vi "Test1_1_ASIC.vi"(4 "Voltages comprobation":dbl[](array[numeric])=[0.05, 0.1, 0.2, 0.5, 0.8, 0.5, 0.6, 0.7, 0.8, 1.0], 7 "Serial Number":string, 8 "error in":errorcluster, 9 "Cycles Burst":i32=10000, 10 "Channels":i32[](array[numeric])=[0, 1, 2, 3, 4, 5, 6], 11 "Instrument VISA in":T1={"AWG VISA"="generadorpulsos", "Oscilloscope  VISA "="Oscilloscope", "Integration Board IP"="172.16.7.43", "connection ID"=refnum, "report out"=refnum, "report file path"=path "C:/Documents and Settings/CTA_LAB01/Desktop/L0_Asic/L0 Asic Test Data"}) -> (0 "error out":errorcluster, 3 "Instrument VISA out":T1={"AWG VISA"="81160A", "Oscilloscope  VISA "="DSO80204B", "Integration Board IP"="172.16.7.43", "connection ID"=refnum, "report out"=refnum, "report file path"=path "C:/Documents and Settings/CTA_LAB01/Desktop/L0_Asic/L0 Asic Test Data"}, 5 "Array":i32[][](array[numeric]))   [LabVIEW 2009]
uses:
  <vilib>/Utility/NIReport.llb/NI_report.lvclass
  <vilib>/Utility/NIReport.llb/HTML/NI_HTML.lvclass
  <instrlib>/Agilent 81150/Agilent 81150.lvlib
  L0_Asic/L0 Asic Test Folder v9/C/Program Files/National Instruments/LabVIEW 2012/instr.lib/Agilent 8000 Series/Agilent 8000 Series.lvlib
  <vilib>/Analysis/NI_AALBase.lvlib
panel:
  in  "Attenuation":i32[](array[numeric])=[0, 4, 10, 12]
  out "Threshold array":i32[](array[numeric])
  out "read buffer 4":string="-1.51468E-08;9.99999E+37;9.99999E+37;1.3964E-09;9.99999E+37;9.99999E+37\n"
  out "report file path":path=path "D:/CTA/Data_test/ASIC/chip_test"
  in  "time to wait":dbl=10.0
  in  "Init values ch":i32[](array[numeric])=[500, 500, 500, 500, 500, 500, 500]
  out "Data output":dbl[][](array[numeric])
  out "time for inner bucle":u32=249
  out "read buffer 3":string
  out "appended array":dbl[](array[numeric])=[1.999998e+38, 0.0, 1.3964e-09, 0.0, 9.99999e+37, 0.0, 9.99999e+37, 0.0, -1.51468e-08, 0.0, 0.0]
  out "points quantity":dbl
  out "Numeric":i32=2147483647
  in  "Save NOW!":bool
  in  "End 2":bool
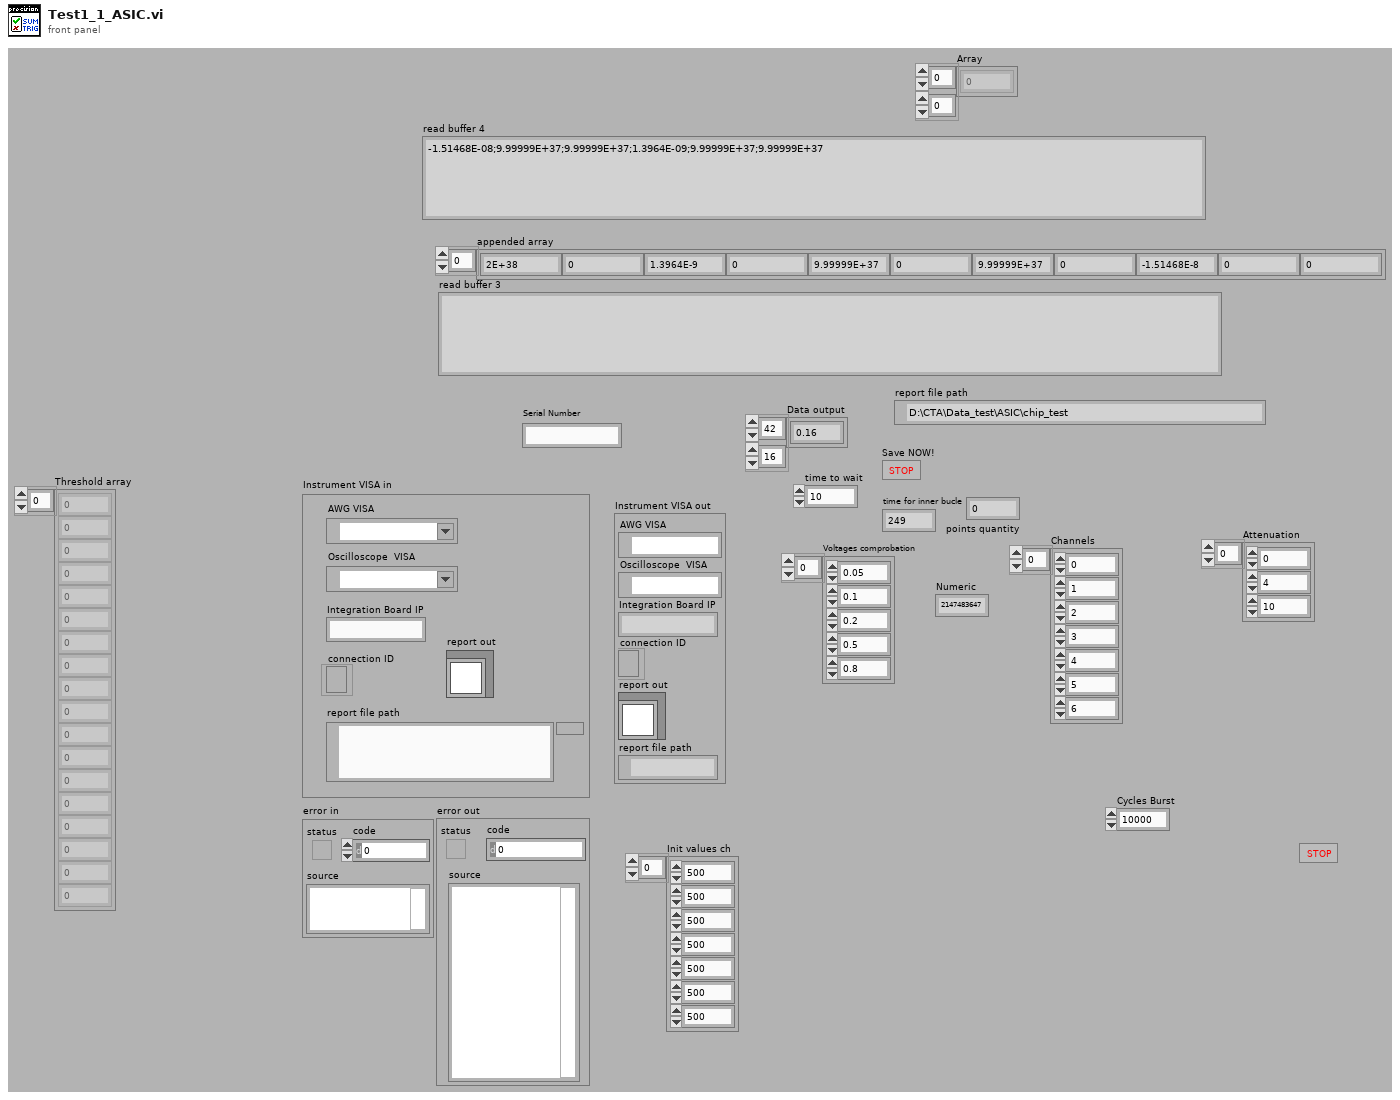
[diagram p1: front panel]
types:
  T1 = cluster{"AWG VISA":refnum<visa-resource-name>, "Oscilloscope  VISA ":refnum<visa-resource-name>, "Integration Board IP":string, "connection ID":refnum<k5>, "report out":refnum<class "NI_report.lvclass">, "report file path":path}
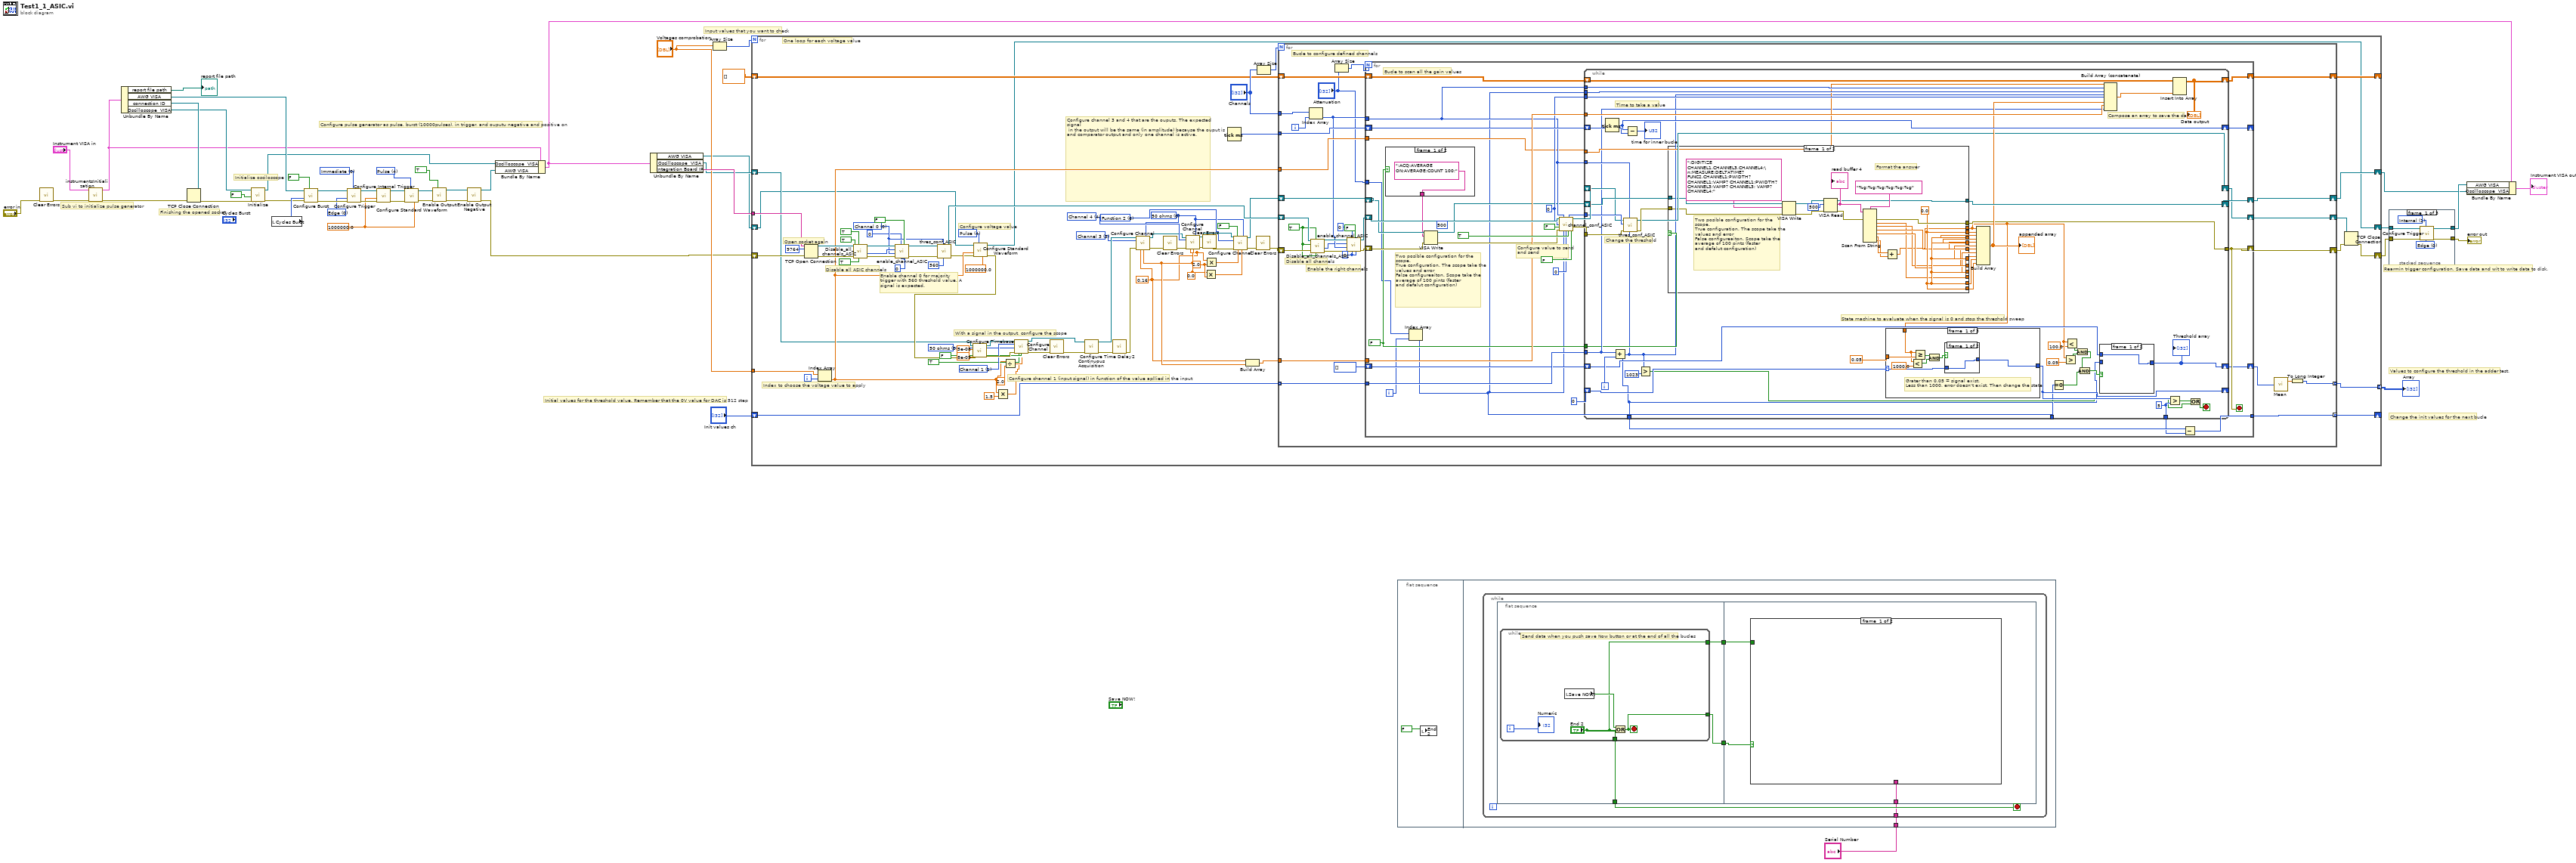
[diagram p0: block diagram]
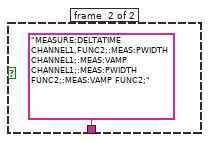
[diagram p2: hidden frame]
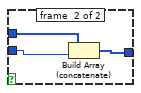
[diagram p3: hidden frame]
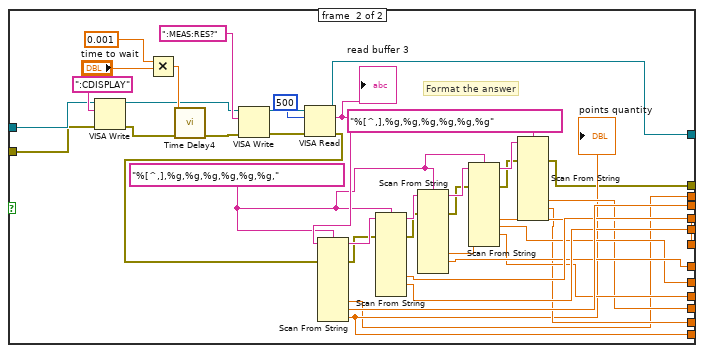
[diagram p4: hidden frame]
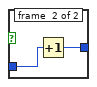
[diagram p5: hidden frame]
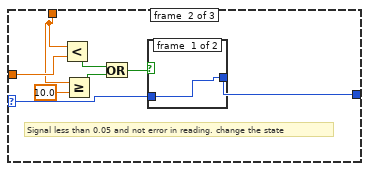
[diagram p6: hidden frame]
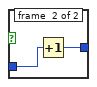
[diagram p7: hidden frame]
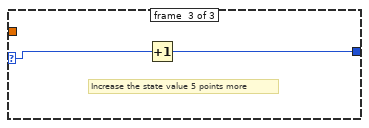
[diagram p8: hidden frame]
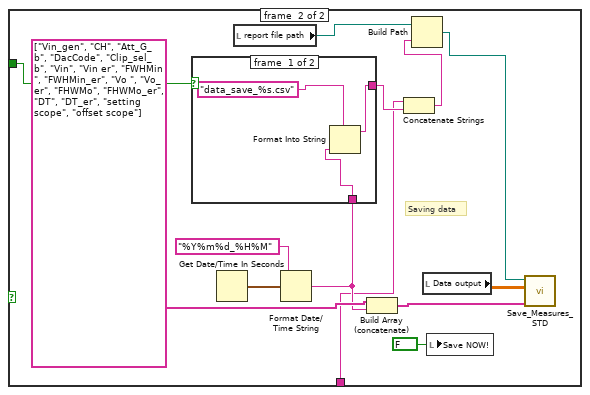
[diagram p9: hidden frame]
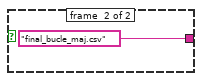
[diagram p10: hidden frame]
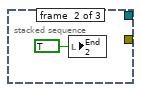
[diagram p11: hidden frame]
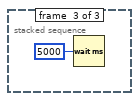
[diagram p12: hidden frame]
diagram:
  w12 = 1000000.0 ("Frequency (1000.0 Hz)")
  w39 = u16 0 items=["Immediate", "Internal", "External", "Software Trigger Function"] ("Trigger Source (0: Immediate)")
  w40 = u16 0 items=["Edge", "Level"] ("Trigger Mode (0: Edge)")
  w44 = u16 4 items=["Sine", "Square", "Ramp Up", "Ramp Down", "Pulse", "Noise", "DC"] ("Waveform (0: Sine)")
  # "Values to configure the threshold in the adder test."
  # "Rearmin trigger configuration. Save data and wit to write data to disk."
  # "Change the init values for the next bucle"
  # "Input values that you want to check"
  # "Initial values for the threshold value. Remember that the 0V value for DAC is 512 step"
  # "Configure pulse generator as pulse, burst (10000pulses), in trigger, and ouputu negative and positive on"
  # "Initialize osciloscope"
  # "Finishing the opened socket"
  # "Sub vi to initialize pulse generator"
  n1 = call <vilib>:"Clear Errors.vi"("error in (no error)"="error in") -> ("error out"=w46:errorcluster)  [unwired: 6 in]
  n2 = call "instrumentsInitialization.vi"("error in"=w46, "Instrument VISA in"="Instrument VISA in") -> ("error out"=w33:errorcluster, "Instrument VISA out"=w24:T1)  [unwired: 8 in]
  n3 = Unbundle By Name(w24) -> ("report file path"=→"report file path":path, "AWG VISA"=w29:refnum<visa-resource-name>, "connection ID"=w34:refnum<k5>, "Oscilloscope  VISA"=w30:refnum<visa-resource-name>)
  n4 = TCP Close Connection(connection ID=w34, error in (no error)=w33) -> (error out=w28:errorcluster)  [unwired: 1 in, 1 out]
  n5 = call "Initialize.vi"("error in (no error)"=w28, "Reset (True)"=FALSE ("ID Query (True)"), "VISA resource name"=w30) -> ("error out"=w8:errorcluster, "VISA resource name out"=w27:refnum<visa-resource-name>)  [unwired: 7 in]
  n6 = local read "Cycles Burst"() -> (w43:i32)
  n7 = call <instrlib>:"Configure Burst.vi"("Enable Burst (F: Disable)"=FALSE, "error in (no error)"=w8, "Burst Count (2)"=w43, "VISA resource name"=w29) -> ("error out"=w42:errorcluster, "VISA resource name out"=w41:refnum<visa-resource-name>)  [unwired: 6 in]
  n8 = call <instrlib>:"Configure Trigger.vi"("Trigger Source (0: Immediate)"=w39, "error in (no error)"=w42, "Trigger Mode (0: Edge)"=w40, "VISA resource name"=w41) -> ("error out"=w38:errorcluster, "VISA resource name out"=w37:refnum<visa-resource-name>)  [unwired: 6 in]
  n9 = call <instrlib>:"Configure Internal Trigger.vi"("error in (no error)"=w38, "Frequency (100000.0 Hz)"=w12, "VISA resource name"=w37) -> ("error out"=w35:errorcluster, "VISA resource name out"=w36:refnum<visa-resource-name>)  [unwired: 7 in]
  n10 = call <instrlib>:"Configure Standard Waveform.vi"("Frequency (1000.0 Hz)"=w12, "Waveform (0: Sine)"=w44, "error in (no error)"=w35, "VISA resource name"=w36) -> ("error out"=w26:errorcluster, "VISA resource name out"=w25:refnum<visa-resource-name>)  [unwired: 6 in]
  n11 = call <instrlib>:"Enable Output.vi"("Enable Output (T: Enable)"=TRUE, "error in (no error)"=w26, "VISA resource name"=w25) -> ("error out"=w11:errorcluster, "VISA resource name out"=w10:refnum<visa-resource-name>)  [unwired: 7 in]
  n12 = call <instrlib>:"Enable Output Negative.vi"("error in (no error)"=w11, "VISA resource name"=w10) -> ("error out"=w2:errorcluster, "VISA resource name out"=w9:refnum<visa-resource-name>)  [unwired: 8 in]
  n13 = Bundle By Name(cluster=w24, "Oscilloscope  VISA"=w27, "AWG VISA"=w9) -> (w7:T1)
  n14 = Unbundle By Name(w7) -> ("AWG VISA"=w5:refnum<visa-resource-name>, "Oscilloscope  VISA"=w6:refnum<visa-resource-name>, "Integration Board IP"=w20:string)
  n15 = Array Size(array="Voltages comprobation") -> (size(s)=w17:i32)
  n16 = for {
    N: w17 -> [_]
    tunnel: w20 -> [w126]
    tunnel: "Voltages comprobation" -> [w125]
    shift-right: [w85] -> _
    shift-left: dbl[][] [] -> [w86]
    shift-right: [w83] -> _
    shift-left: "Init values ch" -> [w84]
    shift-right: [w61] -> w14
    shift-left: w6 -> [w57]
    shift-right: [w127] -> w21
    shift-left: w2 -> [w58]
    shift-right: [w56] -> w13
    shift-left: w5 -> [w50]
    tunnel: [w49] -> w3 mode=indexing
    i -> [w81]
    w62 = 0.16 ("Vertical Range (2.0 V)")
    w63 = 0.0 ("Vertical Offset (0.0 V)")
    w80 = u32 0 ("Clip_sel_b")
    w93 = 2.0 ("y")
    w65 = u32 0 items=["50 ohms", "1 Mohms"] ("Input Impedance (1: 1 Mohms)")
    w73 = u16 0 items=["Channel 0", "Channel 1", "Channel 2", "Channel 3", "Channel 4", "Channel 5", "Channel 6"] ("Channel")
    w113 = u32 0 items=["50 ohms", "1 Mohms"] ("Input Impedance (1: 1 Mohms)")
    w116 = 1 items=["Channel 1"=1, "Channel 2"=2, "Channel 3"=3, "Channel 4"=4] ("Channel (1: Channel 1)")
    w97 = u16 6 items=["Function 1"=5, "Function 2"=6, "Function 3"=7, "Function 4"=8] ("Math Channel (5: Function 1)")
    w64 = 3 items=["Channel 1"=1, "Channel 2"=2, "Channel 3"=3, "Channel 4"=4] ("Channel (1: Channel 1)")
    w111 = 4 items=["Channel 1"=1, "Channel 2"=2, "Channel 3"=3, "Channel 4"=4] ("Channel (1: Channel 1)")
    w123 = u16 4 items=["Sine", "Square", "Ramp Up", "Ramp Down", "Pulse", "Noise", "DC"] ("Waveform (0: Sine)")
    # "Configure channel 3 and 4 that are the ouputs. The expected signal\n in the output will be the same (in amplitude) because the ouput is and comparator output and only one channel is active."
    # "Configure channel 1 (input signal) in function of the value apllied in the input"
    # "With a signal in the output, configure the scope"
    # "Enable channel 0 for majority trigger with 560 threshold value. A signal is expected."
    # "Disable all ASIC channels"
    # "Open socket again"
    # "Configure voltage value"
    # "Index to choose the voltage value to apply"
    # "One loop for each voltage value"
    n17 = TCP Open Connection(address=w126, remote port or service name=u16 9764, error in (no error)=w58) -> (connection ID=w107:refnum<k5>, error out=w106:errorcluster)  [unwired: 2 in]
    n18 = Index Array(array=w125, index=w81) -> (element=w82:dbl)
    n19 = call "Disable_all_channels_ASIC.vi"("CompBuf_en_b"=TRUE, "Att_en_b"=TRUE, "error in"=w106, "Clip_en_b"=TRUE, "connection ID"=w107) -> ("error out"=w105:errorcluster, "id_out"=w103:i32, "connection ID out"=w104:refnum<k5>)  [unwired: 4 in]
    n20 = call "enable_channel_ASIC.vi"("Clip_sel_b"=w80, "maj/sum"=FALSE, "Ib_clipVb"=w80, "Att gain"=u32 0, "error in"=w105, "Channel"=w73, "id_in"=w103, "connection ID"=w104) -> ("error out"=w76:errorcluster, "connection ID out"=w78:refnum<k5>)  [unwired: 1 in, 1 out]
    n21 = call "thres_conf_ASIC.vi"("threshold"=u32 560, "Ring"=w73, "error out 3"=w76, "connection ID"=w78) -> ("error out 2"=w75:errorcluster, "connection ID out"=w77:refnum<k5>)  [unwired: 4 in, 2 out]
    n22 = call <instrlib>:"Configure Standard Waveform.vi"("Frequency (1000.0 Hz)"=1000000.0, "Waveform (0: Sine)"=w123, "error in (no error)"=w75, "Amplitude (1.0 Vpp)"=w82, "VISA resource name"=w50) -> ("error out"=w120:errorcluster, "VISA resource name out"=w56:refnum<visa-resource-name>)  [unwired: 5 in]
    n23 = call "Configure Timebase.vi"("error in (no error)"=w120, "Position (0.0 s)"=8e-09, "Timebase (0.005 s)"=5e-08, "VISA resource name"=w57) -> ("error out"=w117:errorcluster, "VISA resource name out"=w118:refnum<visa-resource-name>)  [unwired: 6 in]
    n24 = Multiply(x=w82, y=1.5) -> (x*y=w94:dbl)
    n25 = Divide(x=w82, y=2.0) -> (x/y=w102:dbl)
    n26 = call "Configure Channel.vi"("VISA resource name"=w118, "Enable Channel (Enable)"=TRUE, "BW Limit 20MHz (Disable)"=FALSE, "Input Impedance (1: 1 Mohms)"=w113, "Channel (1: Channel 1)"=w116, "error in (no error)"=w117, "Vertical Range (2.0 V)"=w94, "Vertical Offset (0.0 V)"=w102) -> ("VISA resource name out"=w53:refnum<visa-resource-name>, "error out"=w115:errorcluster)  [unwired: 6 in]
    n27 = call <vilib>:"Clear Errors.vi"("error in (no error)"=w115) -> ("error out"=w52:errorcluster)  [unwired: 6 in]
    n28 = call "Configure Continuous Acquisition.vi"("error in (no error)"=w52, "VISA resource name"=w53) -> ("error out"=w96:errorcluster, "VISA resource name out"=w66:refnum<visa-resource-name>)  [unwired: 8 in]
    n29 = call "Time Delay2"("error in (no error)"=w96) -> ("error out"=w67:errorcluster)  [unwired: 10 in]
    n30 = call "Configure Channel.vi"("VISA resource name"=w66, "Input Impedance (1: 1 Mohms)"=w65, "Channel (1: Channel 1)"=w64, "error in (no error)"=w67, "Vertical Range (2.0 V)"=w62, "Vertical Offset (0.0 V)"=w63) -> ("VISA resource name out"=w68:refnum<visa-resource-name>, "error out"=w69:errorcluster)  [unwired: 8 in]
    n31 = call <vilib>:"Clear Errors.vi"("error in (no error)"=w69) -> ("error out"=w108:errorcluster)  [unwired: 6 in]
    n32 = call "Configure Channel.vi"("VISA resource name"=w68, "Input Impedance (1: 1 Mohms)"=w65, "Channel (1: Channel 1)"=w111, "error in (no error)"=w108, "Vertical Range (2.0 V)"=w62, "Vertical Offset (0.0 V)"=w63) -> ("VISA resource name out"=w99:refnum<visa-resource-name>, "error out"=w109:errorcluster)  [unwired: 8 in]
    n33 = call <vilib>:"Clear Errors.vi"("error in (no error)"=w109) -> ("error out"=w100:errorcluster)  [unwired: 6 in]
    n34 = Multiply(x=w63, y=w93) -> (x*y=w92:dbl)
    n35 = Multiply(x=w62, y=w93) -> (x*y=w98:dbl)
    n36 = Tick Count (ms)() -> (millisecond timer value=w90:u32)
    n37 = call "Configure Channel.vi"("VISA resource name"=w99, "Enable Channel (Enable)"=FALSE, "Input Impedance (1: 1 Mohms)"=w65, "Channel (1: Channel 1)"=w97, "error in (no error)"=w100, "Vertical Range (2.0 V)"=w98, "Vertical Offset (0.0 V)"=w92) -> ("VISA resource name out"=w60:refnum<visa-resource-name>, "error out"=w101:errorcluster)  [unwired: 7 in]
    n38 = Build Array(w62, w63) -> (w89:dbl[])
    n39 = call <vilib>:"Clear Errors.vi"("error in (no error)"=w101) -> ("error out"=w91:errorcluster)  [unwired: 6 in]
    n40 = Array Size(array="Channels") -> (size(s)=w88:i32)
    n41 = for {
      N: w88 -> [_]
      tunnel: w90 -> [w157]
      tunnel: w89 -> [w156]
      tunnel: "Channels" -> [w155]
      shift-right: [w158] -> w85
      shift-left: w86 -> [w153]
      tunnel: w84 -> [w152] mode=indexing
      tunnel: [w151] -> w83 mode=indexing
      tunnel: w82 -> [w150]
      shift-right: [w149] -> w61
      shift-left: w60 -> [w148]
      shift-right: [w147] -> w59
      shift-left: w91 -> [w144]
      shift-right: [w146] -> w55
      shift-left: w77 -> [w141]
      tunnel: [w130] -> w49 mode=indexing
      i -> [w154]
      w138 = u32 0 ("Ib_clipVb")
      w139 = TRUE ("Att_en_b")
      # "Enable the right channels"
      # "Disable all channels"
      # "Bucle to configure defined channels"
      n42 = Index Array(array=w155, index=w154) -> (element=w136:i32)
      n43 = call "Disable_all_channels_ASIC.vi"("CompBuf_en_b"=w139, "Att_en_b"=w139, "error in"=w144, "Clip_en_b"=w139, "connection ID"=w141) -> ("error out"=w145:errorcluster, "id_out"=w135:i32, "connection ID out"=w142:refnum<k5>)  [unwired: 4 in]
      n44 = Array Size(array="Attenuation") -> (size(s)=w129:i32)
      n45 = call "enable_channel_ASIC.vi"("Clip_sel_b"=w138, "maj/sum"=FALSE, "Ib_clipVb"=w138, "Att gain"=u32 0, "error in"=w145, "Channel"=w136, "id_in"=w135, "connection ID"=w142) -> ("error out"=w143:errorcluster, "connection ID out"=w140:refnum<k5>)  [unwired: 1 in, 1 out]
      n46 = for {
        N: w129 -> [_]
        shift-right: [w185] -> w147
        shift-left: w143 -> [w170]
        shift-right: [w186] -> w158
        shift-left: w153 -> [w193]
        shift-right: [w187] -> w149
        shift-left: w148 -> [w169]
        shift-right: [w179] -> w146
        shift-left: w140 -> [w192]
        tunnel: w156 -> [w190]
        shift-right: [w188] -> _
        shift-left: w157 -> [w189]
        tunnel: w136 -> [w178]
        tunnel: w152 -> [w176]
        tunnel: [w171] -> w151
        tunnel: w150 -> [w174]
        shift-right: [w163] -> w131
        shift-left: i32[] [] -> [w162]
        tunnel: "Attenuation" -> [w161]
        i -> [w160]
        stop <- w185 stop-if-true
        w164 = FALSE
        (unwired) u32 500 ("byte count")
        w180 = u32 0 ("Ib_ClipVb")
        # "Configure value to send and send"
        # "Two posible configuration for the scope. \nTrue configuration. The scope take the values and error\nFalse configureaiton. Scope take the average of 100 pints (faster\nand defalut configuration)"
        # "Bucle to scan all the gain values"
        n47 = case shown="False" w164 {
          tunnel: [":ACQ:AVERAGE ON;AVERAGE:COUNT 100;" ("write buffer") "MEASURE:DELTATIME CHANNEL1,FUNC2;:MEAS:PWIDTH CHANNEL1;:MEAS:VAMP CHANNEL1;:MEAS:PWIDTH FUNC2;:MEAS:VAMP FUNC2;" ("write buffer")] -> w168
          frame #0 {
          }
          frame #1 {
          }
        }
        n48 = Index Array(array=w161, index=w160) -> (element=w159:i32)
        n49 = VISA Write(VISA resource name=w169, write buffer=w168, error in (no error)=w170) -> (VISA resource name out=w166:refnum<visa-resource-name>, error out=w165:errorcluster)  [unwired: 1 out]
        n50 = call "channel_conf_ASIC.vi"("connection ID"=w192, "Ring"=w178, "Clip_sel_b"=w180, "CompBuf_en_b"=FALSE, "error out"=w165, "Att gain"=w159, "Ib_ClipVb"=u32 0, "Clip_en_b"=TRUE, "Att_en_b"=FALSE) -> ("Id out"=w177:i32, "connection ID out"=w167:refnum<k5>, "error out 2"=w182:errorcluster)  [unwired: 2 in, 2 out]
        n51 = while {
          tunnel: w190 -> [w247]
          tunnel: [w230] -> w185
          tunnel: w182 -> [w224]
          tunnel: w180 -> [w228]
          tunnel: w178 -> [w227]
          tunnel: w159 -> [w226]
          tunnel: w178 -> [w222]
          tunnel: w177 -> [w221]
          tunnel: w176 -> [w209]
          shift-right: [w216] -> _
          shift-left: 0 -> [w219]
          tunnel: [w196] -> w173
          tunnel: w174 -> [w217]
          tunnel: [w215] -> w172
          shift-right: [w245] -> w188
          shift-left: w189 -> [w246]
          shift-right: [w243] -> w187
          shift-left: w166 -> [w229]
          shift-right: [w223] -> w179
          shift-left: w167 -> [w214]
          shift-right: [w240] -> w186
          shift-left: w193 -> [w248]
          tunnel: w164 -> [w208]
          shift-right: [w206] -> w163
          shift-left: w162 -> [w205]
          tunnel: w159 -> [w202]
          i -> [w220]
          stop <- w211 stop-if-true
          w215 = 5 ("y")
          # "State machine to evaluate when the signal is 0 and stop the threshold sweep"
          # "Compose an array to save the data"
          # "Change the threshold"
          # "Time to take a value"
          n52 = Tick Count (ms)() -> (millisecond timer value=w245:u32)
          n53 = Add(x=w209, y=w220) -> (x+y=w196:i32)
          n54 = call "thres_conf_ASIC.vi"("threshold"=w196, "Ring"=w222, "error out 3"=w224, "Id in"=w221, "connection ID"=w214) -> ("error out 2"=w225:errorcluster, "connection ID out"=w223:refnum<k5>)  [unwired: 3 in, 2 out]
          n55 = Subtract(x=w245, y=w246) -> (x-y=→"time for inner bucle":u32)
          n56 = Greater?(x=w196, y=1023) -> (0:w210:bool)
          n57 = case shown="False" w208 {
            tunnel: [w267 w301] -> w243
            tunnel: [w265 w300] -> w242
            tunnel: [w261 w293] -> w239
            tunnel: [w265 w292] -> w238
            tunnel: [w262 w291] -> w237
            tunnel: [w265 w290] -> w236
            tunnel: [w260 w289] -> w235
            tunnel: [w265 w288] -> w234
            tunnel: [w259 w287] -> w233
            tunnel: [w265 w286] -> w232
            tunnel: [w265 w285] -> w231
            tunnel: [w266 w283] -> w230
            tunnel: w229 -> [w268 w276]
            tunnel: w225 -> [w257 w274]
            tunnel: [w254 w273] -> w201
            frame #0 {
              w265 = 0.0 ("points quantity")
              # "Format the answer"
              # "Two posible configuration for the scope. \nTrue configuration. The scope take the values and error\nFalse configureaiton. Scope take the average of 100 pints (faster\nand defalut configuration)"
              n58 = VISA Write(VISA resource name=w268, write buffer=":DIGITIZE CHANNEL1,CHANNEL3,CHANNEL4;\n:MEASURE:DELTATIME? FUNC2,CHANNEL1;PWIDTH? CHANNEL1;VAMP? CHANNEL1;PWIDTH? CHANNEL3;VAMP? CHANNEL3; VAMP? CHANNEL4;", error in (no error)=w257) -> (VISA resource name out=w263:refnum<visa-resource-name>, error out=w264:errorcluster)  [unwired: 1 out]
              n59 = VISA Read(VISA resource name=w263, byte count=u32 500, error in (no error)=w264) -> (VISA resource name out=w267:refnum<visa-resource-name>, read buffer=w271:string, error out=w269:errorcluster)  [unwired: 1 out]
              "read buffer 4" <- w271
              n60 = Scan From String(format string="%g;%g;%g;%g;%g;%g", input string=w271, error in=w269) -> (error out=w266:errorcluster, output 1=w259:dbl, output 2=w260:dbl, output 3=w262:dbl, output 4=w261:dbl, output 5=w256:dbl, output 6=w255:dbl)  [unwired: 7 in, 2 out]
              n61 = Add(x=w256, y=w255) -> (x+y=w254:dbl)
            }
            frame #1 {
              w295 = "%[^,],%g,%g,%g,%g,%g,%g," ("format string")
              # "Format the answer"
              n62 = VISA Write(VISA resource name=w276, write buffer=":CDISPLAY", error in (no error)=w274) -> (VISA resource name out=w278:refnum<visa-resource-name>, error out=w275:errorcluster)  [unwired: 1 out]
              n63 = Multiply(x=0.001, y="time to wait") -> (x*y=w303:dbl)
              n64 = call "Time Delay4"("error in (no error)"=w275, "Delay Time (s)"=w303) -> ("error out"=w302:errorcluster)  [unwired: 9 in]
              n65 = VISA Write(VISA resource name=w278, write buffer=":MEAS:RES?", error in (no error)=w302) -> (VISA resource name out=w310:refnum<visa-resource-name>, error out=w309:errorcluster)  [unwired: 1 out]
              n66 = VISA Read(VISA resource name=w310, byte count=u32 500, error in (no error)=w309) -> (VISA resource name out=w301:refnum<visa-resource-name>, read buffer=w306:string, error out=w284:errorcluster)  [unwired: 1 out]
              "read buffer 3" <- w306
              n67 = Scan From String(format string=w295, input string=w306, error in=w284) -> (remaining string=w299:string, error out=w279:errorcluster, output 5=w273:dbl, output 6=w300:dbl, output 7=w285:dbl)  [unwired: 12 in, 1 out]
              "points quantity" <- w285
              n68 = Scan From String(format string=w295, input string=w299, error in=w279) -> (remaining string=w296:string, error out=w280:errorcluster, output 5=w293:dbl, output 6=w292:dbl)  [unwired: 13 in, 1 out]
              n69 = Scan From String(format string=w295, input string=w296, error in=w280) -> (remaining string=w297:string, error out=w281:errorcluster, output 5=w291:dbl, output 6=w290:dbl)  [unwired: 13 in, 1 out]
              n70 = Scan From String(format string=w295, input string=w297, error in=w281) -> (remaining string=w298:string, error out=w282:errorcluster, output 5=w289:dbl, output 6=w288:dbl)  [unwired: 13 in, 1 out]
              n71 = Scan From String(format string="%[^,],%g,%g,%g,%g,%g,%g", input string=w298, error in=w282) -> (error out=w283:errorcluster, output 5=w287:dbl, output 6=w286:dbl)  [unwired: 13 in, 2 out]
            }
          }
          n72 = case shown="2, Default" w219 {
            selector: w219 -> [w311 w322 w333]
            tunnel: [w318 w328 w334] -> w216
            tunnel: w201 -> [w316 w323 _]
            tunnel: 0.05 ("y") -> [w317 w329 _]
            frame #0 {
              # "Grater than 0.05 = signal exist.\nLess than 1000, error doesn't exist. Then change the state"
              n73 = Less?(x=w316, y=1000.0) -> (x < y?=w312:bool)
              n74 = Greater Or Equal?(x=w316, y=w317) -> (x >= y?=w313:bool)
              n75 = And(x=w313, y=w312) -> (x .and. y?=w314:bool)
              n76 = case shown="True" w314 {
                tunnel: w311 -> [w319 w321]
                tunnel: [w319 w320] -> w318
                frame #0 {
                }
                frame #1 {
                  n77 = Increment(x=w321) -> (x+1=w320:i32)
                }
              }
            }
            frame #1 {
              # "Signal less than 0.05 and not error in reading. change the state"
              n78 = Less?(x=w323, y=w329) -> (x < y?=w326:bool)
              n79 = Greater Or Equal?(x=w323, y=10.0) -> (x >= y?=w325:bool)
              n80 = Or(x=w326, y=w325) -> (x .or. y?=w327:bool)
              n81 = case shown="False" w327 {
                tunnel: w322 -> [w330 w332]
                tunnel: [w330 w331] -> w328
                frame #0 {
                }
                frame #1 {
                  n82 = Increment(x=w332) -> (x+1=w331:i32)
                }
              }
            }
            frame #2 {
              # "Increase the state value 5 points more"
              n83 = Increment(x=w333) -> (x+1=w334:i32)
            }
          }
          n84 = Build Array(w201, w242, w239, w238, w237, w236, w235, w234, w233, w232, w231) -> (w241:dbl[])
          "appended array" <- w241
          n85 = Equal To 0?(x=w202) -> (x = 0?=w203:bool)
          n86 = Greater?(x=w201, y=0.09) -> (0:w198:bool)
          n87 = Less?(x=w201, y=100.0) -> (x < y?=w199:bool)
          n88 = And(x=w199, y=w198) -> (x .and. y?=w197:bool)
          n89 = And(x=w197, y=w203) -> (x .and. y?=w204:bool)
          n90 = case shown="True" w204 {
            tunnel: w196 -> [_ w253]
            tunnel: w205 -> [w250 w252]
            tunnel: [w250 w251] -> w206
            frame #0 {
            }
            frame #1 {
              n91 = Build Array (concatenate)(w252, w253) -> (w251:i32[])
            }
          }
          "Threshold array" <- w206
          n92 = Build Array (concatenate)(w217, w227, w226, w196, w228, w241, w247, w209) -> (w249:dbl[])
          n93 = Greater?(x=w216, y=w215) -> (0:w212:bool)
          n94 = Insert Into Array(array=w248, new element=w249) -> (w240:dbl[][])  [unwired: 2 in]
          "Data output" <- w240
          n95 = Or(x=w212, y=w210) -> (x .or. y?=w211:bool)
        }
        n96 = Subtract(x=w173, y=w172) -> (x-y=w171:i32)
      }
      n97 = call <vilib>:"Mean.vi"("X"=w131) -> ("mean"=w132:dbl)  [unwired: 1 out]
      n98 = To Long Integer(number=w132) -> (32bit integer=w130:i32)
    }
    n99 = TCP Close Connection(connection ID=w55, error in (no error)=w59) -> (error out=w127:errorcluster)  [unwired: 1 in, 1 out]
  }
  "Array" <- w3
  n100 = flat-sequence {
    tunnel: "Serial Number" -> [w336]
    frame #0 {
      n101 = local write "End 2"(FALSE ("End")) -> ()
    }
    frame #1 {
      n102 = while {
        tunnel: w336 -> [w337]
        stop <- w338 stop-if-true
        n103 = flat-sequence {
          tunnel: [w343] -> w340
          tunnel: [w342] -> w339
          tunnel: [w341] -> w338
          tunnel: w340 -> [w350]
          tunnel: w339 -> [w349]
          tunnel: w337 -> [w348]
          frame #0 {
            n104 = while {
              tunnel: [w346] -> w343
              tunnel: ["End 2"] -> w342
              tunnel: ["End 2"] -> w341
              i -> [w345]
              stop <- w346 stop-if-true
              # "Send data when you push save Now button or at the end of all the bucles"
              n105 = local read "Save NOW!"() -> (w347:bool)
              n106 = Or(x=w347, y="End 2") -> (x .or. y?=w346:bool)
              "Numeric" <- w345
            }
          }
          frame #1 {
            n107 = case shown="True" w350 {
              tunnel: w349 -> [_ w360]
              tunnel: w348 -> [_ w351]
              frame #0 {
              }
              frame #1 {
                # "Saving data"
                n108 = Get Date/Time In Seconds() -> (seconds since 1Jan1904=w357:timestamp)
                n109 = local read "report file path"() -> (w362:path)
                n110 = Format Date/Time String(time format string (%c)="%Y%m%d_%H%M", seconds (now)=w357) -> (date/time string=w355:string)  [unwired: 1 in]
                n111 = case shown="True" w360 {
                  tunnel: [w365 "final_bucle_maj.csv" ("format string")] -> w352
                  tunnel: w355 -> [w364 _]
                  frame #0 {
                    n112 = Format Into String(format string="data_save_%s.csv", w364) -> (resulting string=w365:string)  [unwired: 2 in, 1 out]
                  }
                  frame #1 {
                  }
                }
                n113 = Build Array (concatenate)(string[] ["Vin_gen", "CH", "Att_G_b", "DacCode", "Clip_sel_b", "Vin", "Vin er", "FWHMin ", "FWHMin_er", "Vo ", "Vo_er", "FHWMo", "FHWMo_er", "DT", "DT_er", "setting scope", "offset scope"] ("appended array"), w355) -> (w358:string[])
                n114 = Concatenate Strings(w351, w352) -> (w353:string)
                n115 = Build Path(base path=w362, name or relative path=w353) -> (appended path=w363:path)
                n116 = local read "Data output"() -> (w354:dbl[][])
                n117 = local write "Save NOW!"(FALSE ("Save NOW!")) -> ()
                n118 = call "Save_Measures_STD.vi"("appended array"=w358, "Data in"=w354, "file path (dialog if empty)"=w363) -> ()  [unwired: 9 in]
              }
            }
          }
        }
      }
    }
  }
  n119 = stacked-sequence {
    tunnel: w21 -> [w371 _ _]
    tunnel: [w370 _ _] -> w4
    tunnel: w13 -> [w369 _ _]
    tunnel: [w368 _ _] -> w15
    frame #0 {
      w372 = u16 1 items=["Immediate", "Internal", "External", "Software Trigger Function"] ("Trigger Source (0: Immediate)")
      w373 = u16 0 items=["Edge", "Level"] ("Trigger Mode (0: Edge)")
      n120 = call <instrlib>:"Configure Trigger.vi"("Trigger Source (0: Immediate)"=w372, "error in (no error)"=w371, "Trigger Mode (0: Edge)"=w373, "VISA resource name"=w369) -> ("error out"=w370:errorcluster, "VISA resource name out"=w368:refnum<visa-resource-name>)  [unwired: 6 in]
    }
    frame #1 {
      n121 = local write "End 2"(TRUE ("End 2")) -> ()
    }
    frame #2 {
      n122 = Wait (ms)(milliseconds to wait=u32 5000) -> ()  [unwired: 1 out]
    }
  }
  "error out" <- w4
  n123 = Bundle By Name(cluster=w7, "AWG VISA"=w15, "Oscilloscope  VISA"=w14) -> (→"Instrument VISA out":T1)
